vi "publish -- set -- 7.vi"(8 "request event":refnum<user-event>, 9 "response ref":refnum<vi>, 10 "data":cluster{"a":dbl, "b":dbl, "c":cdb}) -> ()   [LabVIEW 2018]
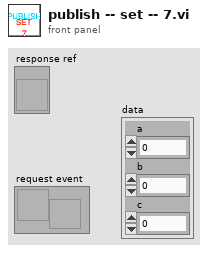
[diagram p1: front panel]
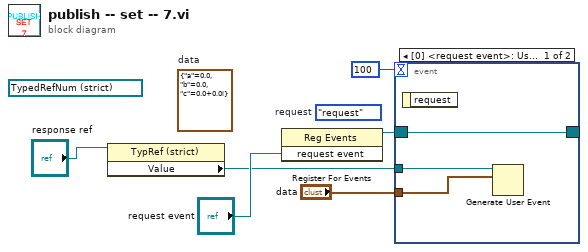
[diagram p0: block diagram]
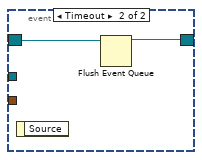
[diagram p2: hidden frame]
diagram:
  (unwired) refnum<vi> refnum ("response ref")
  (unwired) cluster{"a":dbl, "b":dbl, "c":cdb} {"a"=0.0, "b"=0.0, "c"=0.0+0.0i}  # data
  (unwired) enum16{"request"}."request"  # request
  n1 = property class="TypRef (strict)"(reference="response ref") -> ("Value"=w1:refnum<user-event>)  [unwired: 1 in, 2 out]
  n2 = register-events("request event") -> (reference out=w6:refnum<event-registration>)  [unwired: 2 in, 1 out]
  n3 = event shown="[0] <request event>: User Event" {
    selector: w6 -> [w9 w11]
    dyn-events: [w9 w10] -> _
    timeout: 100 -> [_ _]
    tunnel: w1 -> [w8 _]
    tunnel: "data" -> [w7 _]
    event User Event {
      n4 = event-data() -> ()  [unwired: 1 in, 1 out]
      n5 = Generate User Event(user event=w8, event data cluster=w7) -> ()  [unwired: 2 in, 2 out]
    }
    event Timeout {
      n6 = event-data() -> ()  [unwired: 1 in, 1 out]
      n7 = Flush Event Queue(0:w11) -> (8:w10:refnum<event-registration>)  [unwired: 5 in, 2 out]
    }
  }
